vi "String_to String 2D Array.vi"(9 "Seperators Column ()":string[](array[string]), 10 "Seperators Row (\\n)":string[](array[string]), 11 "Input String":string="MM,MS-XX|MA_SM\nMS,AM-XM|SM_SA\nAM,XS-XM|AA_MM\nMS,AM-AS|MS_MX\nXM,AS-AM|XA_MM\nXX,AM-MX|XA_MA\nSM,SM-SA|SX_SS\nSA,XA-MA|SA_AA\nMA,MM-MX|MM_MM\nMX,MX-AX|MA_SX") -> (3 "2D Array":string[][](array[string]))   [LabVIEW 2025]
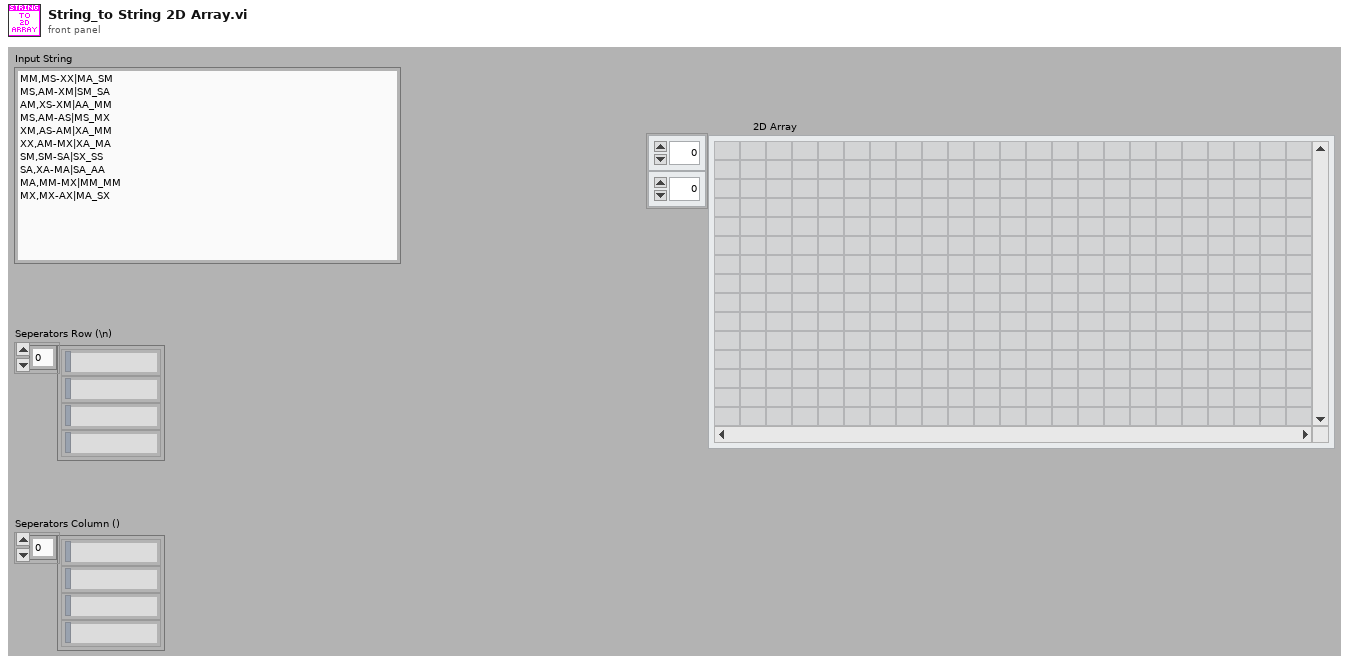
[diagram p1: front panel]
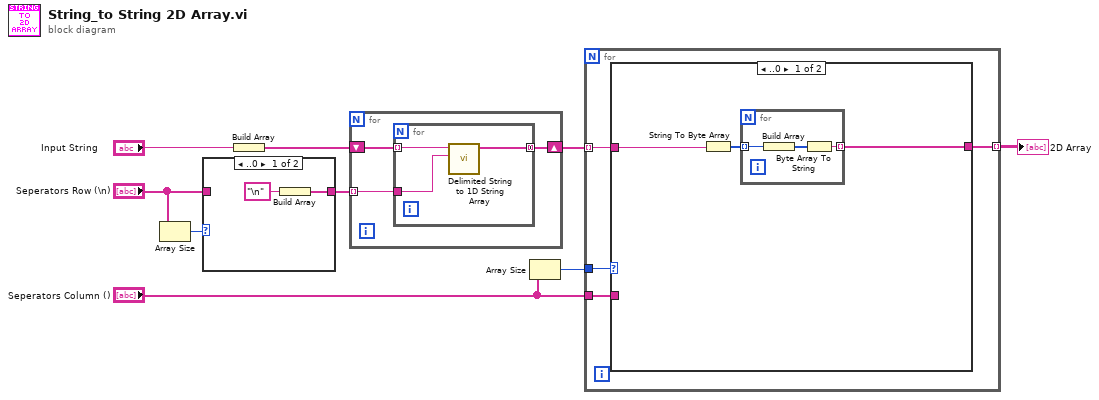
[diagram p0: block diagram]
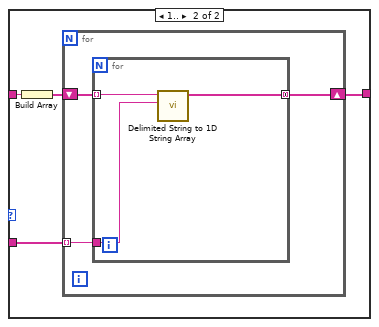
[diagram p2: hidden frame]
diagram:
  n1 = Array Size(array="Seperators Row (\\n)") -> (size(s)=w8:i32)
  n2 = case shown="..0" w8 {
    tunnel: [w10 w12] -> w7
    tunnel: "Seperators Row (\\n)" -> [_ w12]
    frame ..0 {
      n3 = Build Array("\n" ("delimiter")) -> (w10:string[])
    }
    frame 1.. {
    }
  }
  n4 = Build Array("Input String") -> (w5:string[])
  n5 = for {
    tunnel: w7 -> [w14] mode=indexing
    shift-right: [w13] -> w4
    shift-left: w5 -> [w15]
    n6 = for {
      tunnel: w15 -> [w18] mode=indexing
      tunnel: w14 -> [w17]
      tunnel: [w16] -> w13 mode=concatenating
      n7 = call <vilib>:"Delimited String to 1D String Array.vi"("delimiter"=w17, "delimited string"=w18) -> ("string array"=w16:string[])  [unwired: 9 in]
    }
  }
  n8 = Array Size(array="Seperators Column ()") -> (size(s)=w2:i32)
  n9 = for {
    tunnel: w4 -> [w21] mode=indexing
    tunnel: "Seperators Column ()" -> [w19]
    tunnel: w2 -> [w22]
    tunnel: [w20] -> w1 mode=indexing
    n10 = case shown="..0" w22 {
      tunnel: w21 -> [w25 w31]
      tunnel: [w23 w29] -> w20
      tunnel: w19 -> [_ w32]
      frame ..0 {
        n11 = String To Byte Array(string=w25) -> (unsigned byte array=w24:u8[])
        n12 = for {
          tunnel: w24 -> [w28] mode=indexing
          tunnel: [w26] -> w23 mode=indexing
          n13 = Build Array(w28) -> (w27:u8[])
          n14 = Byte Array To String(unsigned byte array=w27) -> (string=w26:string)
        }
      }
      frame 1.. {
        n15 = Build Array(w31) -> (w30:string[])
        n16 = for {
          tunnel: w32 -> [w34] mode=indexing
          shift-right: [w33] -> w29
          shift-left: w30 -> [w35]
          n17 = for {
            tunnel: w35 -> [w38] mode=indexing
            tunnel: w34 -> [w37]
            tunnel: [w36] -> w33 mode=concatenating
            n18 = call <vilib>:"Delimited String to 1D String Array.vi"("delimiter"=w37, "delimited string"=w38) -> ("string array"=w36:string[])  [unwired: 9 in]
          }
        }
      }
    }
  }
  "2D Array" <- w1
